vi "Load Signal Bank (TC).vi"(4 "error in (no error)":errorcluster, 5 "Input array":dbl[][](array[numeric])=array10000x1[10000 elements] format="%.2f", 6 "Active AO Array":i32[](array[numeric]), 7 "timeout (ms)":i32=5000) -> (0 "error out":errorcluster={"status"=FALSE, "code"=0, "source"="."})   [LabVIEW 2015]
uses:
  DAQ Engine VIs/PXI Globals.vi
panel:
  out "Waveform Graph":dbl[][](graph)
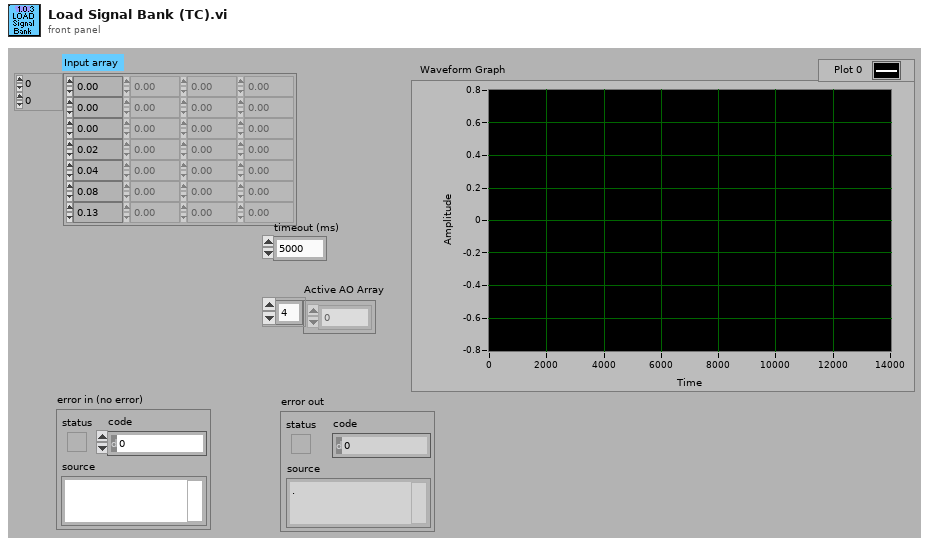
[diagram p1: front panel]
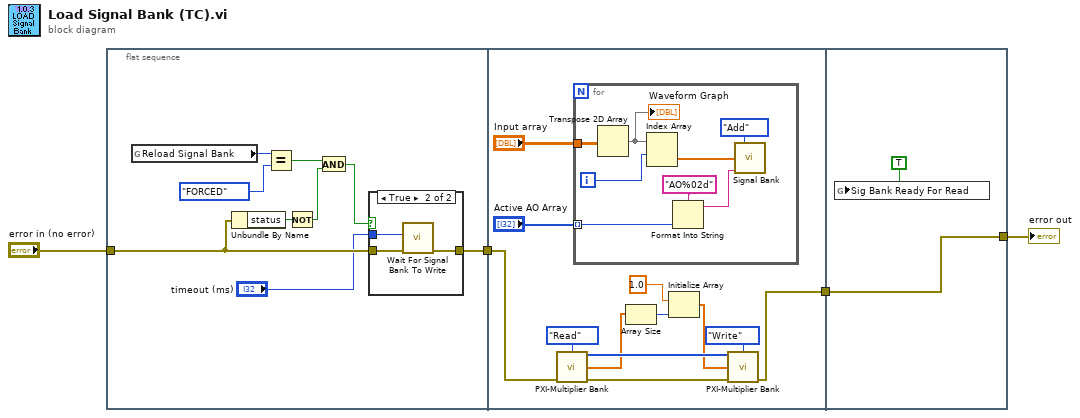
[diagram p0: block diagram]
diagram:
  n1 = flat-sequence {
    tunnel: "error in (no error)" -> [w6]
    tunnel: [w13] -> w3
    tunnel: w3 -> [w29]
    tunnel: [w23] -> w2
    tunnel: [w38] -> w1
    tunnel: w2 -> [w38]
    frame #0 {
      n2 = global read "PXI Globals.vi" "Reload Signal Bank"() -> (w8:enum32{"OFF", "ENABLED", "FORCED"})
      n3 = Unbundle By Name(w6) -> ("status"=w10:bool)
      n4 = Equal?(x=w8, y=enum16{"OFF", "ENABLED", "FORCED"}."FORCED") -> (x = y?=w12:bool)
      n5 = Not(x=w10) -> (.not. x?=w11:bool)
      n6 = And(x=w12, y=w11) -> (x .and. y?=w7:bool)
      n7 = case shown="True" w7 {
        tunnel: w6 -> [w14 w17]
        tunnel: [w14 w16] -> w13
        tunnel: "timeout (ms)" -> [_ w15]
        frame False {
        }
        frame True {
          n8 = call "Wait For Signal Bank To Write.vi"("error in (no error)"=w17, "timeout (ms)"=w15) -> ("error out"=w16:errorcluster)  [unwired: 8 in, 1 out]
        }
      }
    }
    frame #1 {
      n9 = call "PXI-Multiplier Bank.vi"("Action"=enum16{"Init", "Write", "Read"}."Read", "error in (no error)"=w29) -> ("Channels"=w20:i32[], "Multipliers out"=w19:dbl[], "error out"=w24:errorcluster)  [unwired: 11 in]
      n10 = for {
        tunnel: "Active AO Array" -> [w36] mode=indexing
        tunnel: "Input array" -> [w31]
        i -> [w34]
        n11 = Transpose 2D Array(2D array=w31) -> (transposed array=w30:dbl[][])
        "Waveform Graph" <- w30
        n12 = Index Array(array=w30, index (row)=w34) -> (element=w33:dbl[])  [unwired: 1 in]
        n13 = Format Into String(format string="AO%02d", w36) -> (resulting string=w35:string)  [unwired: 2 in, 1 out]
        n14 = call "Signal Bank.vi"("Action"=enum16{"Add", "Replace ID", "Read ID", "Clear"}."Add", "1D Data In"=w33, "ID"=w35) -> ()  [unwired: 11 in, 2 out]
      }
      n15 = Array Size(array=w19) -> (size(s)=w26:i32)
      n16 = Initialize Array(1.0 ("element"), w26) -> (w18:dbl[])
      n17 = call "PXI-Multiplier Bank.vi"("AO Channels"=w20, "Action"=enum16{"Init", "Write", "Read"}."Write", "Multipliers"=w18, "error in (no error)"=w24) -> ("error out"=w23:errorcluster)  [unwired: 9 in, 2 out]
    }
    frame #2 {
      n18 = global write "PXI Globals.vi" "Sig Bank Ready For Read"(TRUE) -> ()
    }
  }
  "error out" <- w1
